vi "Update Sink Level.vi"(8 "error in (no error)":errorcluster, 10 "LogLevel":T1, 11 "Log Sink":refnum<data-value>) -> (0 "error out":errorcluster)   [LabVIEW 2017, in "Composed Log.lvlib" / "Log Sink.lvclass"]
uses:
  <vilib>/gpm_packages/@cs/event-logger/Source/Composed Log/Log Sink/Log Sink.lvclass
  <vilib>/gpm_packages/@cs/event-logger/Source/Composed Log/Types/Log Level.ctl
  <vilib>/gpm_packages/@cs/event-logger/Source/Composed Log/Log Sink/Log Sink.lvclass/Log Sink.ctl
  <vilib>/gpm_packages/@cs/event-logger/Source/Composed Log/Composed Log.lvlib
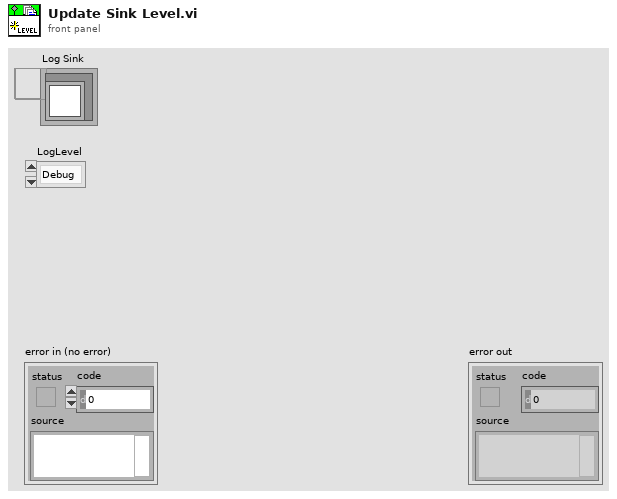
[diagram p1: front panel]
types:
  T1 = typedef "Composed Log.lvlib/Log Level.ctl" = enum16{"Debug", "Info", "Warning", "Error", "Critical"}
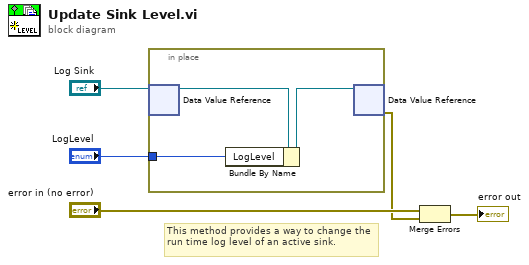
[diagram p0: block diagram]
diagram:
  # "This method provides a way to change the run time log level of an active sink."
  n1 = in-place {
    in-place-border: "LogLevel" -> [w6]
    n2 = in-place-dvr #1("Log Sink") -> (w8:refnum<class "Log Sink.lvclass">)  [unwired: 1 out]
    n3 = Bundle By Name(cluster=w8, "LogLevel"=w6) -> (w7:refnum<class "Log Sink.lvclass">)
    n4 = in-place-dvr #1(w7) -> (w1:errorcluster)  [unwired: 1 out]
  }
  n5 = Merge Errors("error in (no error)", w1) -> (→"error out":errorcluster)
